vi "gentonos.vi"() -> ()   [LabVIEW 2020]
uses:
  <vilib>/Analysis/3filter.llb/FIR Filter (DBL).vi
  <vilib>/Analysis/NI_AALBase.lvlib
panel:
  in  "L ventana":i32
  out "Waveform Graph":dbl[](graph)
  in  "f2":dbl=0.1 format="%#_13g"
  in  "f1":dbl=0.1 format="%#_13g"
  in  "FFT size":i32=-1
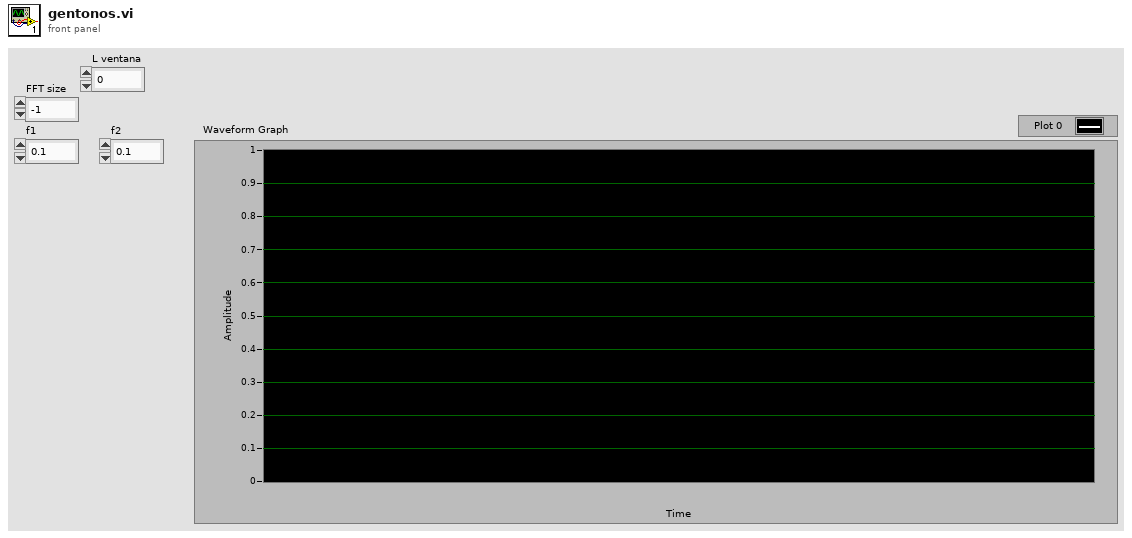
[diagram p1: front panel]
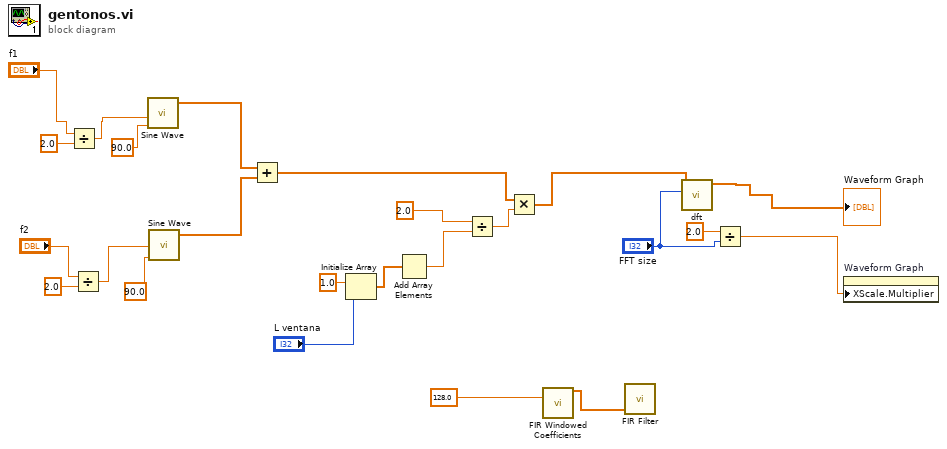
[diagram p0: block diagram]
diagram:
  n1 = Divide(x="f1", y=2.0) -> (x/y=w14:dbl)
  n2 = Divide(x="f2", y=2.0) -> (x/y=w11:dbl)
  n3 = call <vilib>:"Sine Wave.vi"("frequency"=w14, "phase in"=90.0) -> ("sine wave"=w18:dbl[])  [unwired: 3 in, 2 out]
  n4 = call <vilib>:"Sine Wave.vi"("frequency"=w11, "phase in"=90.0) -> ("sine wave"=w17:dbl[])  [unwired: 3 in, 2 out]
  n5 = Add(x=w18, y=w17) -> (x+y=w4:dbl[])
  n6 = Initialize Array(1.0 ("element"), "L ventana") -> (w7:dbl[])
  n7 = Add Array Elements(numeric array=w7) -> (sum=w6:dbl)
  n8 = Divide(x=2.0, y=w6) -> (x/y=w5:dbl)
  n9 = Multiply(x=w4, y=w5) -> (x*y=w3:dbl[])
  n10 = call <vilib>:"FIR Windowed Coefficients.vi"("sampling freq: fs"=128.0) -> ("FIR Windowed Coefficients"=w2:dbl[])  [unwired: 13 in, 1 out]
  n11 = call-poly <vilib>:"FIR Filter.vi"("FIR Coefficients"=w2) -> ()  [unwired: 3 in, 2 out]
  n12 = call "dft.vi"("FFT size"="FFT size", "X"=w3) -> ("FFT X"=→"Waveform Graph":dbl[])  [unwired: 9 in]
  n13 = Divide(x=2.0, y="FFT size") -> (x/y=w20:dbl)
  n14 = property on="Waveform Graph" class="WFGraph (strict)"("XScale.Multiplier"=w20) -> ()  [unwired: 2 in, 2 out]
